vi "1L19_demo_temp.vi"(4 "error in (no error)":errorcluster) -> (0 "error out":errorcluster, 3 "temp":dbl format="%.2f")   [LabVIEW 2010, in "lv_01.lvlib"]
uses:
  lv_01.lvlib
panel:
  in  "Readings":dbl[](array[numeric])=[163.0, 163.0, 163.0, 163.0, 163.0, 163.0, 165.0, 169.0, 172.0, 173.0, 172.0, 172.0, 171.0, 171.0, 174.0, 176.0, 177.0, 178.0, 178.0, 179.0, 178.0, 177.0, 176.0, 175.0, 175.0, 174.0, 173.0, 172.0, 172.0, 172.0, 172.0, 172.0, 171.0, 171.0, 170.0, 170.0, 170.0, 172.0, 173.0, 174.0, 175.0, 177.0, 178.0, 178.0, 178.0, 177.0, 176.0, 175.0, 176.0, 178.0, 179.0, 180.0, 179.0, 178.0, 178.0, 176.0, 176.0, 176.0, 174.0, 174.0, 174.0, 173.0, 173.0, 175.0, 176.0, 178.0, 178.0, 177.0, 176.0, 175.0, 175.0, 174.0, 174.0, 173.0, 173.0, 172.0, 172.0, 171.0, 171.0, 170.0, 170.0, 170.0, 170.0, 170.0, 170.0, 170.0, 169.0, 166.0, 167.0, 169.0, 170.0, 169.0, 168.0, 168.0, 168.0, 168.0, 167.0, 167.0, 167.0, 167.0] format="%.2f"
  # "*This VI is a demo version of a \nVI that reads the voltage on\nDevice 1, channel 0 and scales\nthe signal by 100 to convert to\ntemperature.*"
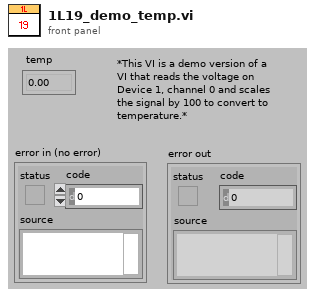
[diagram p1: front panel]
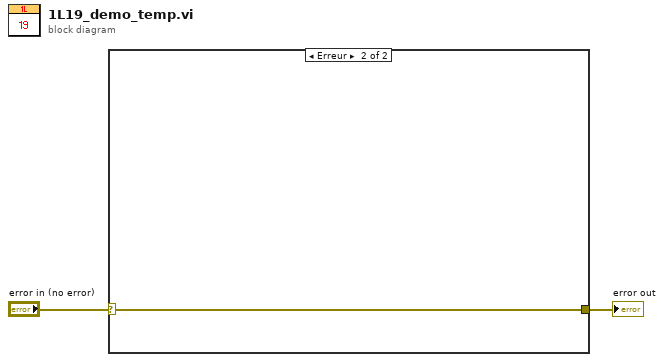
[diagram p0: block diagram]
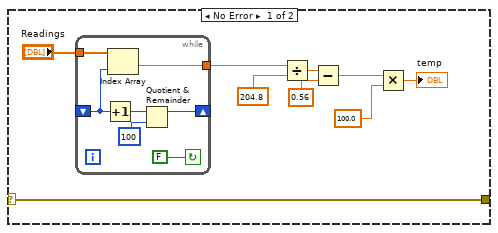
[diagram p2: hidden frame]
diagram:
  n1 = case shown="Erreur" "error in (no error)" {
    selector: "error in (no error)" -> [w6 w19]
    tunnel: [w6 w19] -> w1
    frame No Error {
      n2 = while {
        tunnel: "Readings" -> [w13]
        tunnel: [w14] -> w9
        shift-left: _ -> [w18]
        shift-right: [w15] -> _
        stop <- FALSE continue-if-true
        n3 = Increment(x=w18) -> (x+1=w17:i32)
        n4 = Index Array(array=w13, index=w18) -> (element=w14:dbl)
        n5 = Quotient & Remainder(x=w17, y=100) -> (x-y*floor(x/y)=w15:i32)  [unwired: 1 out]
      }
      n6 = Divide(x=w9, y=204.8) -> (x/y=w8:dbl)
      n7 = Subtract(x=w8, y=0.56) -> (x-y=w4:dbl)
      n8 = Multiply(x=w4, y=100.0) -> (x*y=→"temp":dbl)
    }
    frame Error {
    }
  }
  "error out" <- w1
